vi "Main.vi"() -> ()   [LabVIEW 2019]
uses:
  States.ctl
  <vilib>/ErrorRing/Error Ring.xnode
panel:
  in  "stop":bool
  out "WPM":u32
  out "Letter Count":u32
  out "Word Count":i32
  in  "UserInput":string
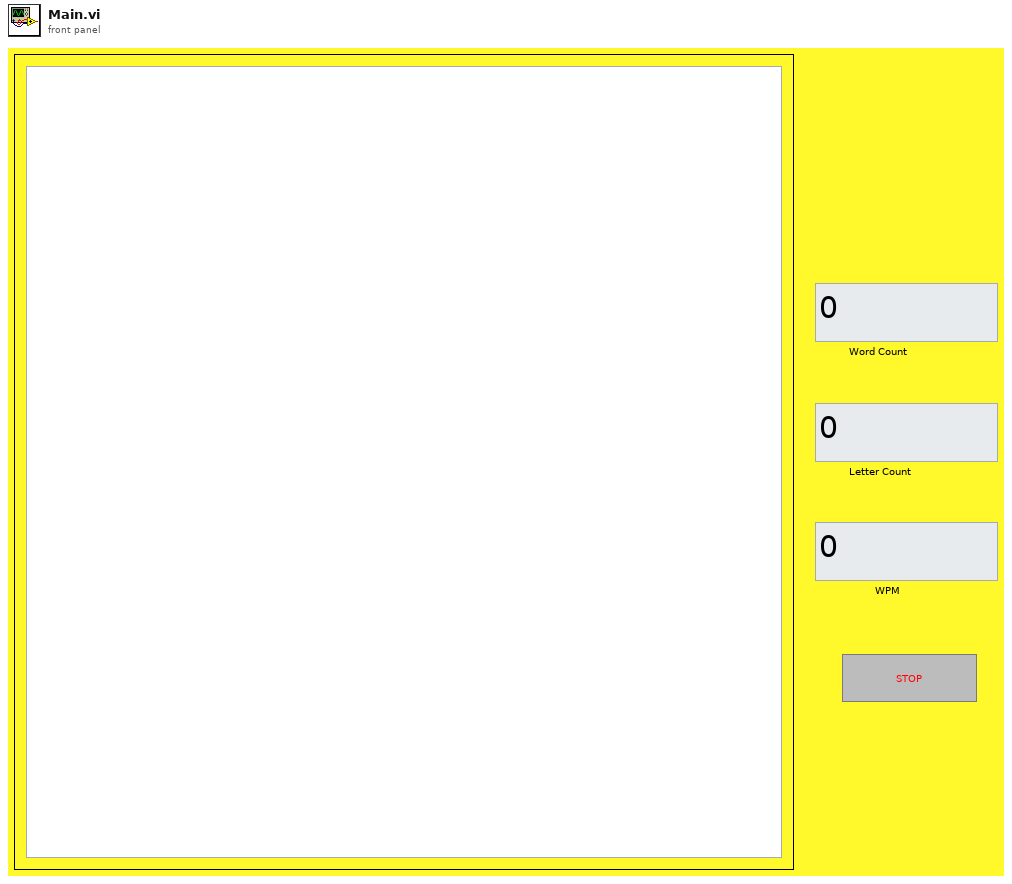
[diagram p1: front panel]
types:
  T1 = typedef "States.ctl" = enum16{"Idle", "Data Initialize", "UI Initialize", "UIUpdate", "CalculateStringLength", "CalculateTypingSpeed", "CalculateWordLimit", "MacroExit", "Exit"}
  T2 = cluster{"This VI":refnum<vi>, "TimeOut":i32, "UserEnteredString":string, "StringLength":u32, "millisecond timer value":u32, "TimeArray":u32[], "TypingSpeed":u32, "WordCount":i32}
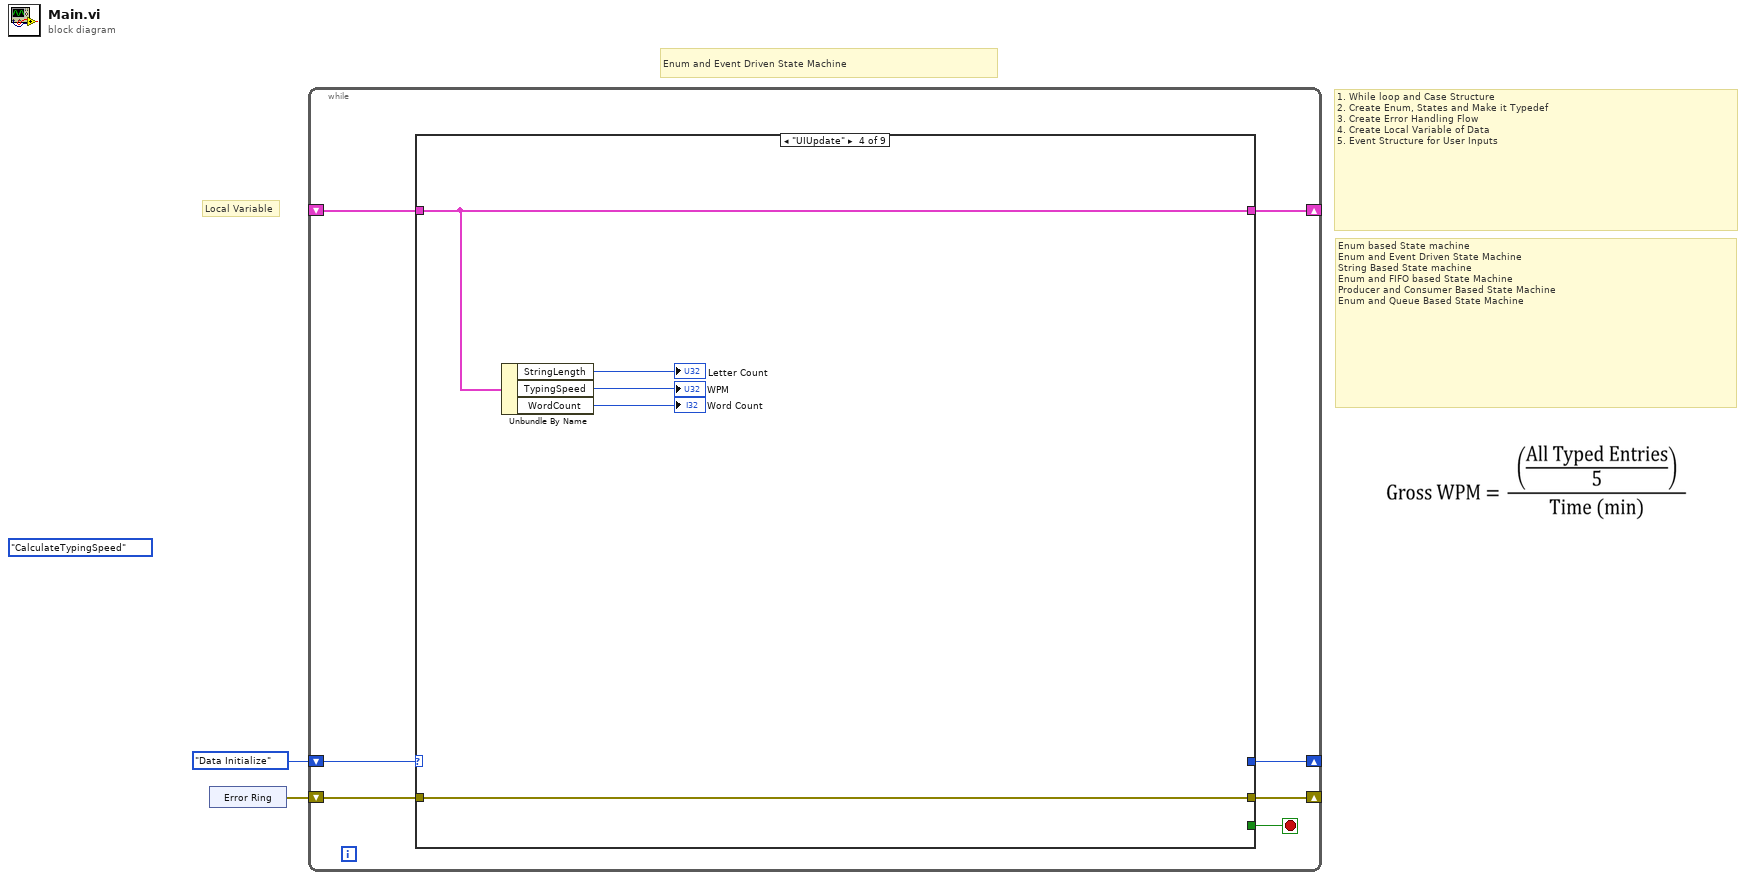
[diagram p0: block diagram]
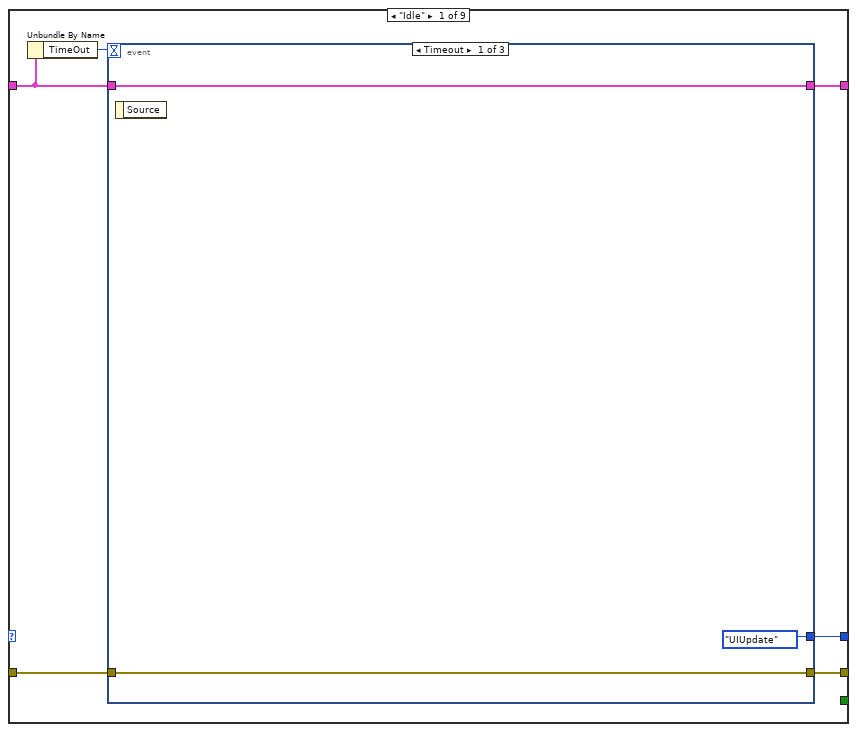
[diagram p2: hidden frame]
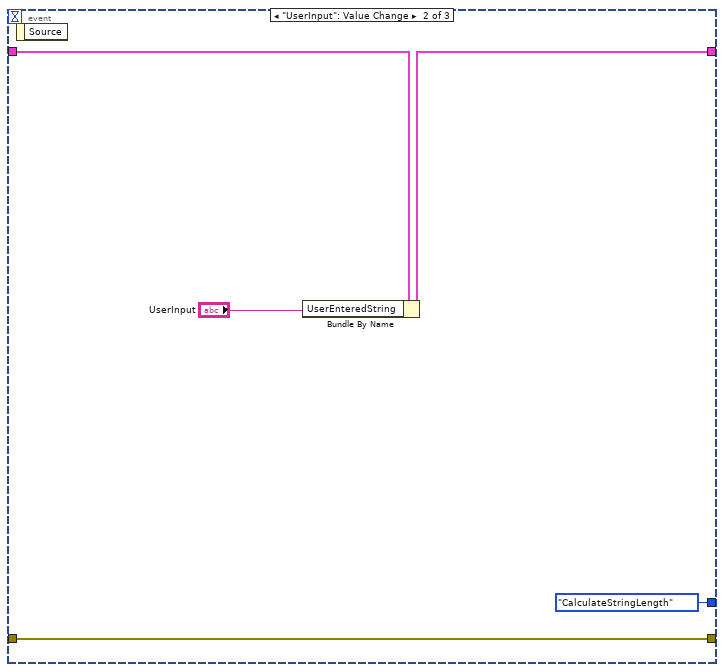
[diagram p3: hidden frame]
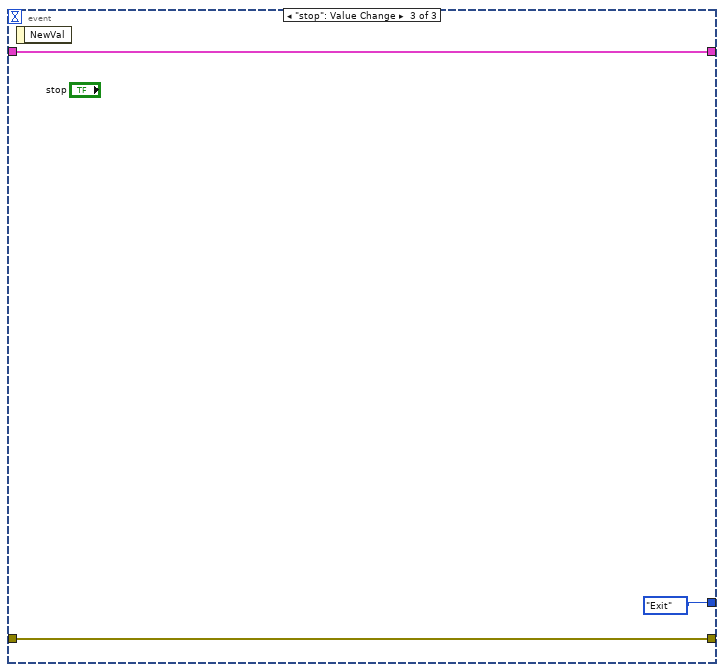
[diagram p4: hidden frame]
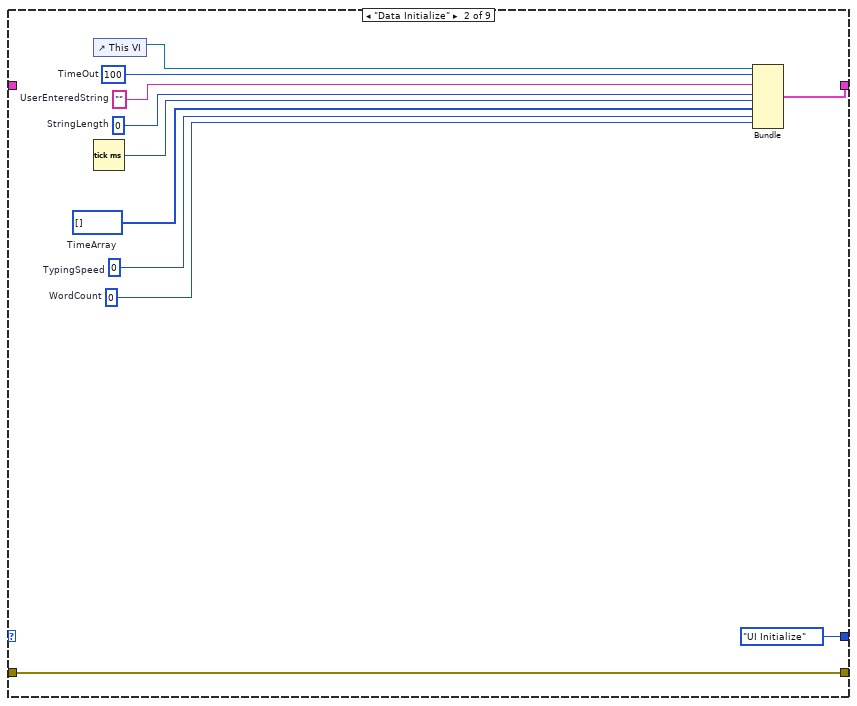
[diagram p5: hidden frame]
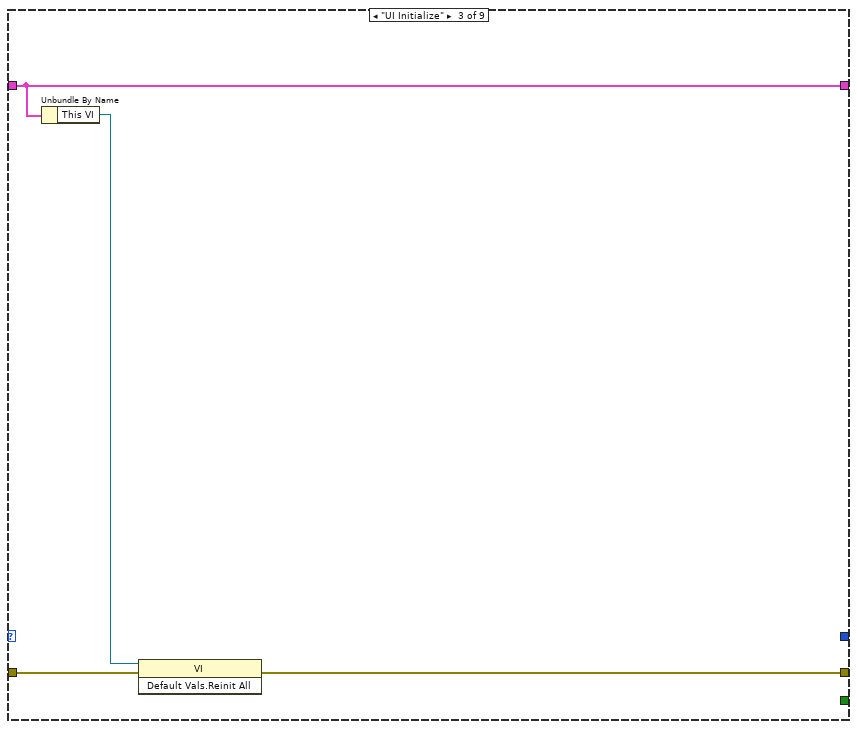
[diagram p6: hidden frame]
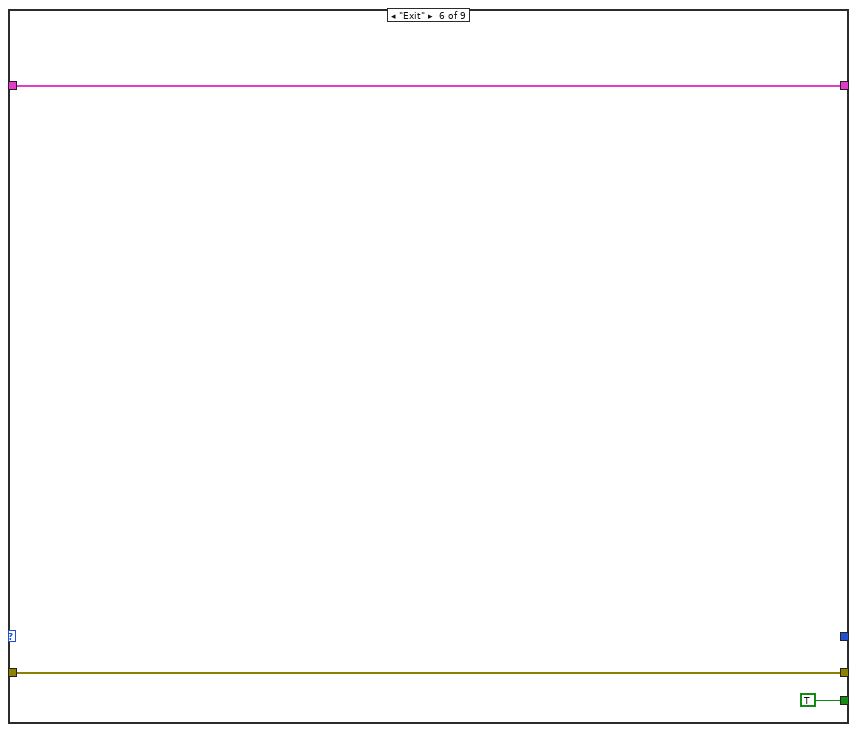
[diagram p8: hidden frame]
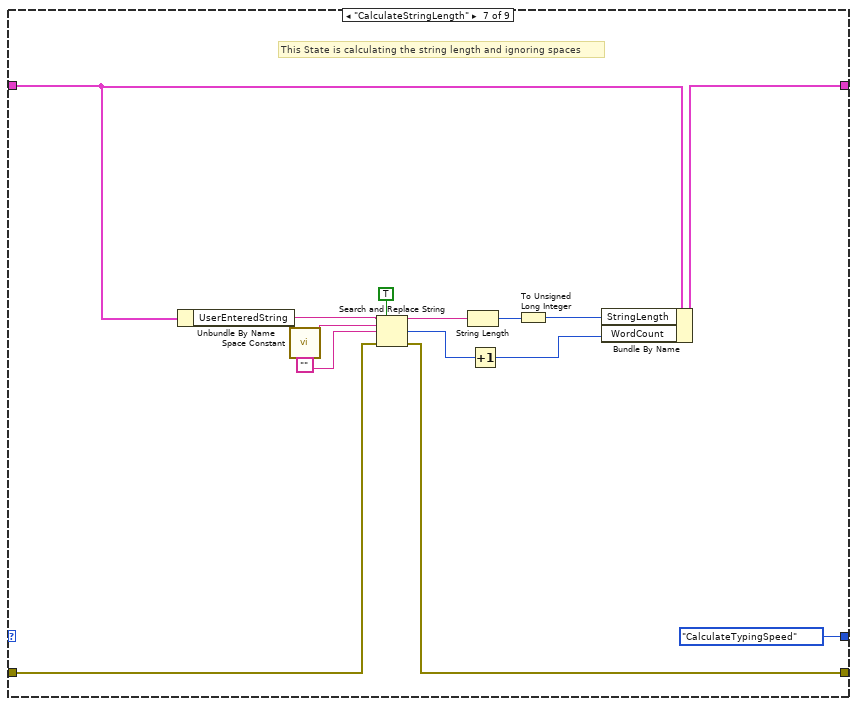
[diagram p9: hidden frame]
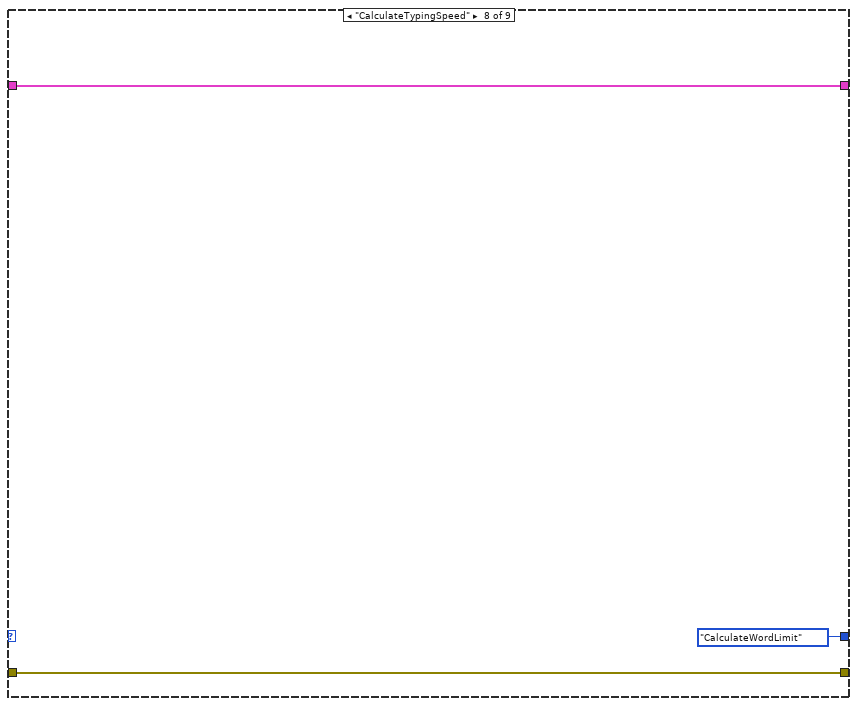
[diagram p10: hidden frame]
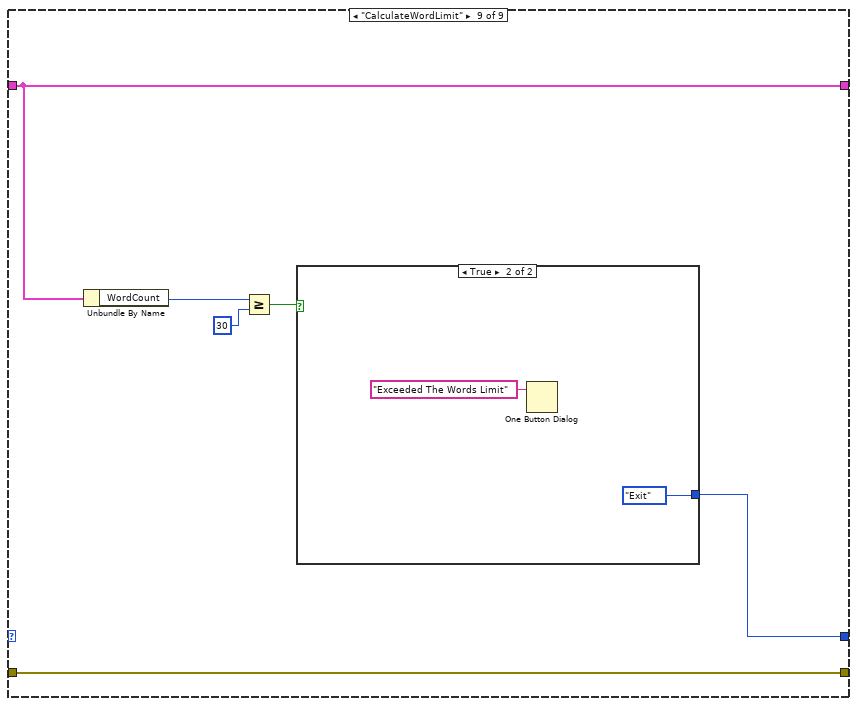
[diagram p11: hidden frame]
diagram:
  (unwired) States."CalculateTypingSpeed"
  # "Local Variable"
  # "1. While loop and Case Structure\n2. Create Enum, States and Make it Typedef\n3. Create Error Handling Flow\n4. Create Local Variable of Data\n5. Event Structure for User Inputs"
  # "Enum and Event Driven State Machine"
  # "Enum based State machine\nEnum and Event Driven State Machine\nString Based State machine\nEnum and FIFO based State Machine\nProducer and Consumer Based State Machine\nEnum and Queue Based State Machine"
  n1 = xnode "Error Ring"() -> ("error out"=w1:errorcluster)
  n2 = while {
    shift-right: [w4] -> _
    shift-left: States."Data Initialize" -> [w9]
    shift-right: [w7] -> _
    shift-left: w1 -> [w8]
    shift-right: [w6] -> _
    shift-left: _ -> [w5]
    stop <- w3 stop-if-true
    n3 = case shown="\"UIUpdate\"" w9 {
      tunnel: w8 -> [w15 w37 w38 w46 w48 w51 w57 w68 w74]
      tunnel: [w14 w37 w39 w46 w48 w51 w58 w68 w74] -> w7
      tunnel: [w13 w36 w41 w45 w47 w50 w64 w67 w71] -> w6
      tunnel: w5 -> [w12 _ w41 w45 w47 w50 w63 w67 w71]
      tunnel: [w10 States."UI Initialize" _ _ _ _ States."CalculateTypingSpeed" States."CalculateWordLimit" w69] -> w4
      tunnel: [_ _ _ _ _ TRUE _ _ _] -> w3
      frame "Idle" {
        n4 = Unbundle By Name(w12) -> ("TimeOut"=w11:i32)
        n5 = event shown="[0] Timeout" {
          selector: _ -> [_ _ _]
          dyn-events: _ -> [_ _ _]
          timeout: w11 -> [_ _ _]
          tunnel: w15 -> [w18 w23 w26]
          tunnel: [w18 w23 w26] -> w14
          tunnel: w12 -> [w17 w19 w25]
          tunnel: [w17 w22 w25] -> w13
          tunnel: [States."UIUpdate" States."CalculateStringLength" States."Exit"] -> w10
          event Timeout {
            n6 = event-data() -> ()  [unwired: 1 in, 1 out]
          }
          event "UserInput": Value Change {
            n7 = event-data() -> ()  [unwired: 1 in, 1 out]
            n8 = Bundle By Name(cluster=w19, "UserEnteredString"="UserInput") -> (w22:T2)
          }
          event "stop": Value Change {
            n9 = event-data() -> ()  [unwired: 1 in, 1 out]
          }
        }
      }
      frame "Data Initialize" {
        w27 = 0  # WordCount
        w29 = u32 0  # TypingSpeed
        w30 = u32[] []  # TimeArray
        w33 = u32 0  # StringLength
        w34 = ""  # UserEnteredString
        w35 = 100  # TimeOut
        n10 = control-ref of="This VI"() -> (w32:refnum<vi>)
        n11 = Tick Count (ms)() -> (millisecond timer value=w28:u32)
        n12 = Bundle("This VI"=w32, "TimeOut"=w35, "UserEnteredString"=w34, "StringLength"=w33, "millisecond timer value"=w28, "TimeArray"=w30, "TypingSpeed"=w29, "WordCount"=w27) -> (w36:T2)  [unwired: 1 in]
      }
      frame "UI Initialize" {
        n13 = Unbundle By Name(w41) -> ("This VI"=w40:refnum<vi>)
        n14 = invoke class="VI" method="Default Vals.Reinit All"(reference=w40, error in=w38) -> (error out=w39:errorcluster)  [unwired: 1 in, 2 out]
      }
      frame "UIUpdate" {
        n15 = Unbundle By Name(w45) -> ("StringLength"=→"Letter Count":u32, "TypingSpeed"=→"WPM":u32, "WordCount"=→"Word Count":i32)
      }
      frame "MacroExit" {
      }
      frame "Exit" {
      }
      frame "CalculateStringLength" {
        # "This State is calculating the string length and ignoring spaces"
        n16 = Unbundle By Name(w63) -> ("UserEnteredString"=w62:string)
        n17 = call <vilib>:"Space Constant.vi"() -> ("String"=w61:string)
        n18 = Search and Replace String(replace all?=TRUE ("replace all? (F)"), input string=w62, search string=w61, replace string="", error in=w57) -> (result string=w56:string, number of replacements=w53:i32, error out=w58:errorcluster)  [unwired: 3 in, 1 out]
        n19 = String Length(string=w56) -> (length=w65:i32)
        n20 = Increment(x=w53) -> (x+1=w52:i32)
        n21 = To Unsigned Long Integer(number=w65) -> (unsigned 32bit integer=w55:u32)
        n22 = Bundle By Name(cluster=w63, "StringLength"=w55, "WordCount"=w52) -> (w64:T2)
      }
      frame "CalculateTypingSpeed" {
      }
      frame "CalculateWordLimit" {
        n23 = Unbundle By Name(w71) -> ("WordCount"=w72:i32)
        n24 = Greater Or Equal?(x=w72, y=30) -> (x >= y?=w70:bool)
        n25 = case shown="True" w70 {
          tunnel: [_ States."Exit"] -> w69
          frame False {
          }
          frame True {
            n26 = One Button Dialog(message="Exceeded The Words Limit") -> ()  [unwired: 1 in, 1 out]
          }
        }
      }
    }
  }
